vi "Export Strings.vi"(4 "error in":errorcluster, 5 "Log File":path, 6 "String File":path, 7 "Target":path) -> (0 "error out":errorcluster, 1 "Log File Out":path, 2 "String File Out":path)   [LabVIEW 2025]
doc: "This VI exports all strings of a single VI or of all elements in a LabVIEW Project to a file using the <b>VIs Strings.Export</b> invoke method. Additionally, the histories of all VIs and the descriptions of the project and of any libraries (classes) are added to the exported file.\n\nThe provided target <b>must</b> have the extension <i>.lvproj</i> or <i>.vi</i>.\n\nThe path input <b>Log File</b> is passed only to the <b>VIs Strings.Export</b> invoke method and has no further usage.\n\nThe <b>String File</b> and <b>Log File</b> inputs are optional. If they are not provided the files will be saved to a temporary location. The used paths are represented by the correspondent outputs."
uses:
  Type Definitions/Export Strings States--enum.ctl
  Type Definitions/Export Strings Data--enum.ctl
  Type Definitions/Extensions--enum.ctl
  Type Definitions/Project References--cluster.ctl
  <vilib>/Utility/EditLVProj/Library And VI References.ctl
  <userlib>/_OpenG.lib/file/file.llb/Strip Path Extension - Path__ogtk.vi
  <userlib>/_OpenG.lib/file/file.llb/Strip Path - Traditional__ogtk.vi
  <userlib>/_OpenG.lib/file/file.llb/File Exists - Scalar__ogtk.vi
  <vilib>/Utility/EditLVProj/Edit LVProj.lvlib
  <userlib>/_OpenG.lib/file/file.llb/openg_file.lvlib
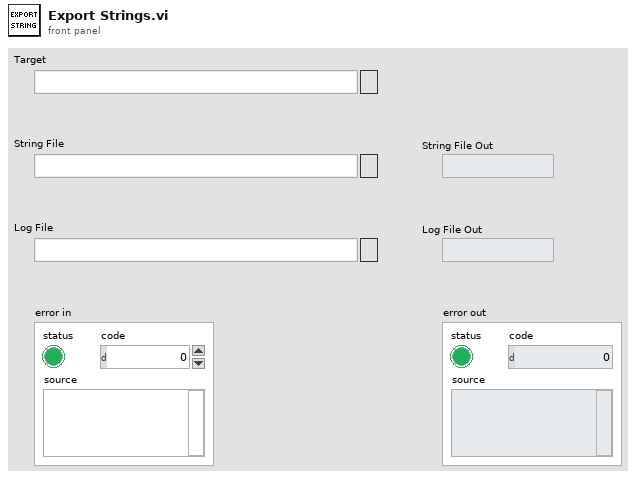
[diagram p1: front panel]
types:
  T1 = typedef "Export Strings Data--enum.ctl" = cluster{"Extension":T2, "String File":path, "Log File":path, "All VIs":refnum<vi>[], "All Libraries":refnum<vi>[], "Reference":variant}
  T2 = typedef "Extensions--enum.ctl" = enum16{"lvproj", "vi"}
  T3 = typedef "Export Strings States--enum.ctl" = enum16{"Initialize", "Exit", "Export Strings", "Export Project Desc.", "Remove Files", "Export VI Histories", "Export Libraries Desc.", "Prepare VI", "Prepare Project", "Create Folders"}
  T4 = typedef "Project References--cluster.ctl" = cluster{"Project Ref":refnum<vi>, "VI-Lib Ref":T5[]}
  T5 = typedef "Edit LVProj.lvlib/Library And VI References.ctl" = cluster{"Target Reference":refnum<vi>, "VI References":refnum<vi>[], "Library References":refnum<vi>[]}
  T6 = enum16{"open", "replace", "create", "open or create", "replace or create", "replace or create with confirmation"}
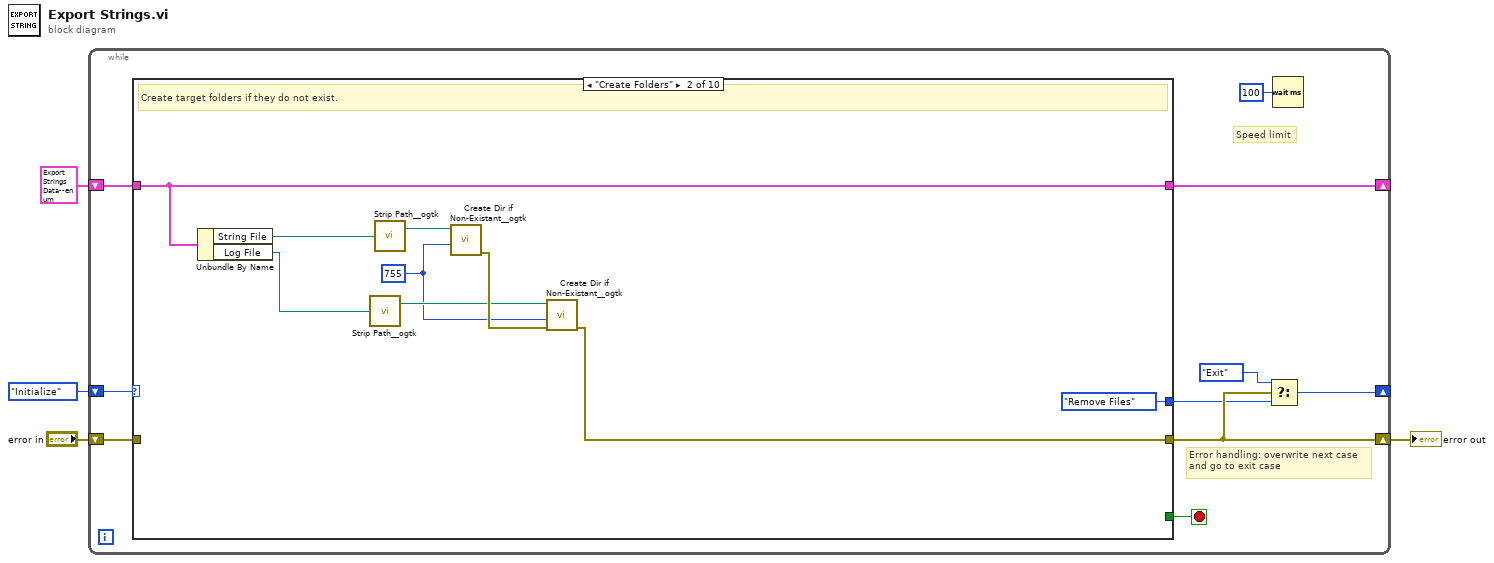
[diagram p0: block diagram]
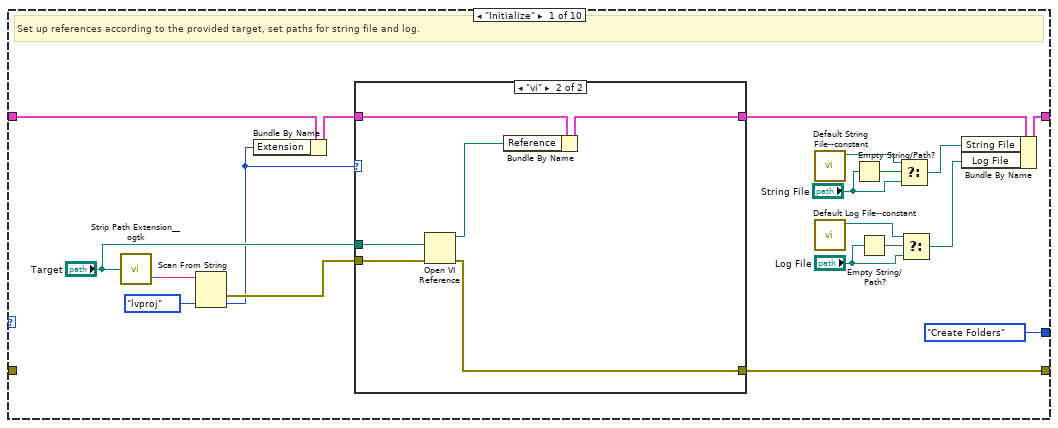
[diagram p2: hidden frame]
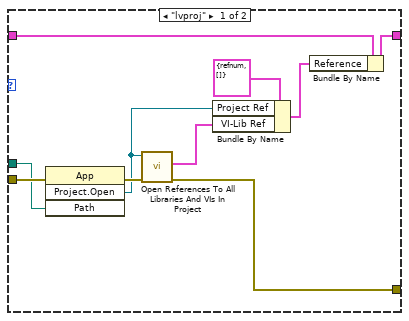
[diagram p3: hidden frame]
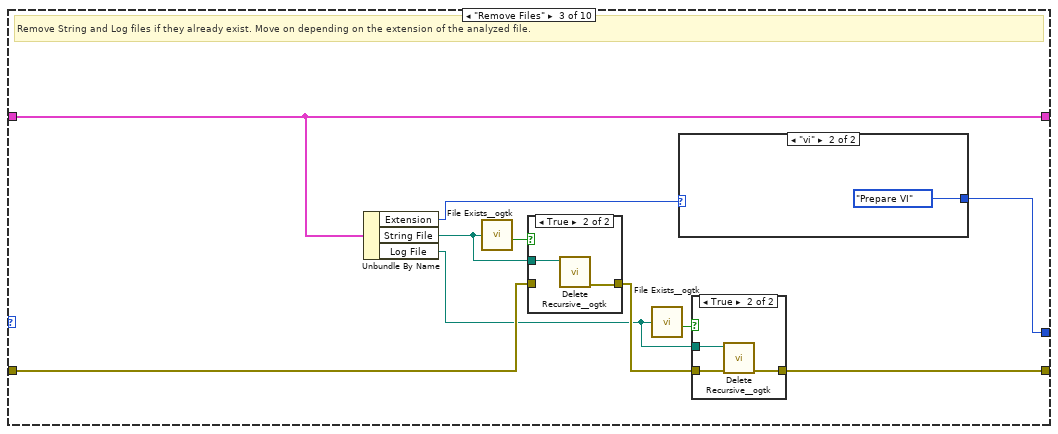
[diagram p4: hidden frame]
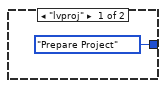
[diagram p5: hidden frame]
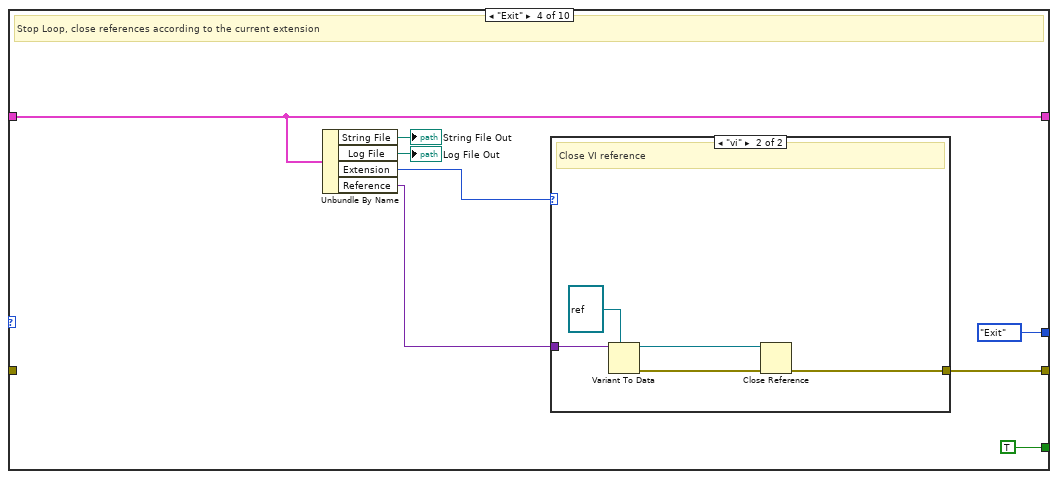
[diagram p8: hidden frame]
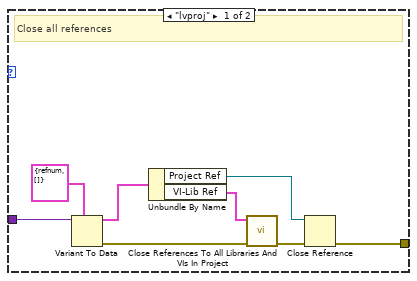
[diagram p9: hidden frame]
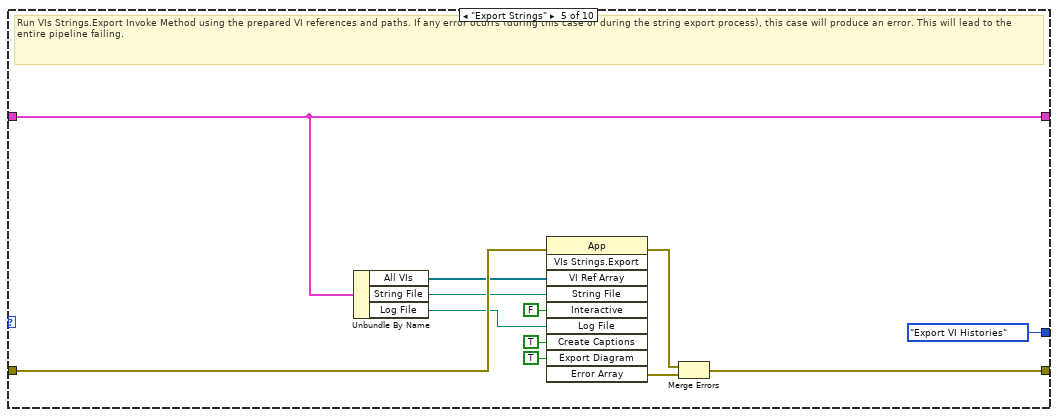
[diagram p10: hidden frame]
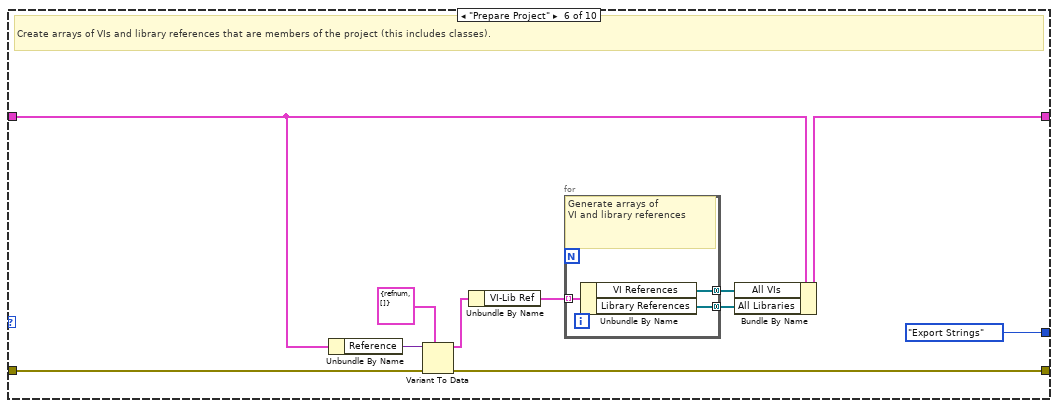
[diagram p11: hidden frame]
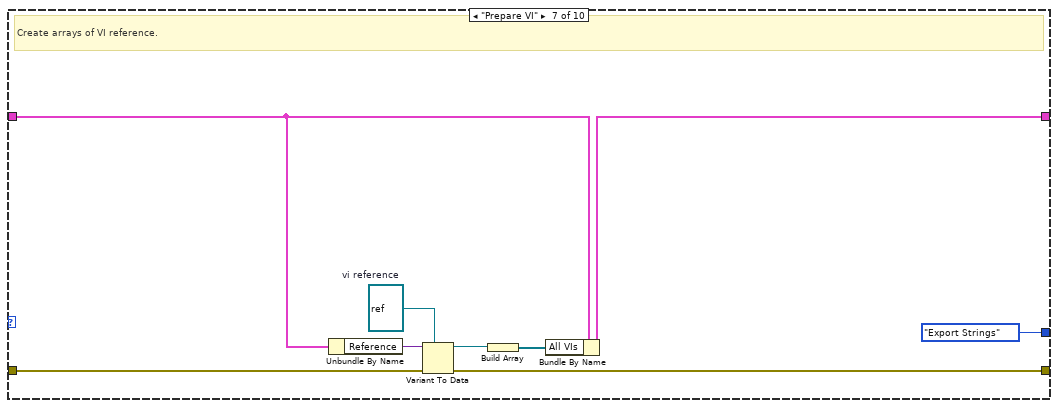
[diagram p12: hidden frame]
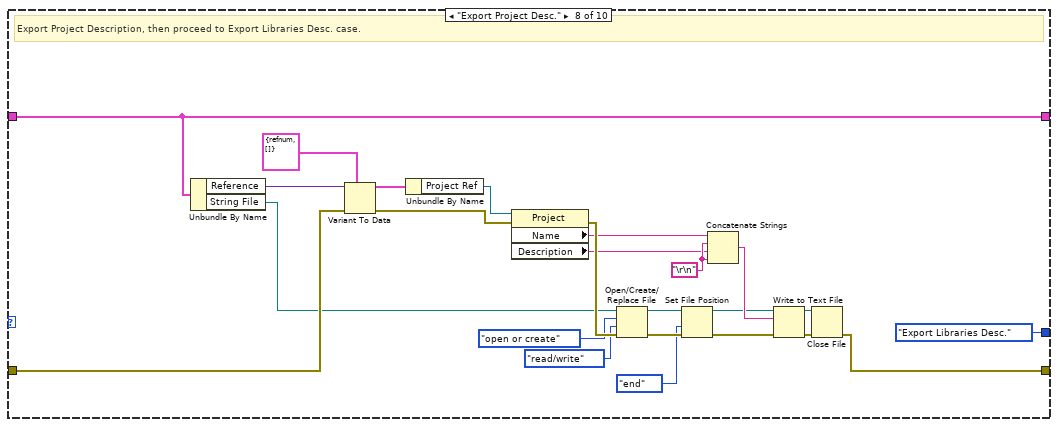
[diagram p13: hidden frame]
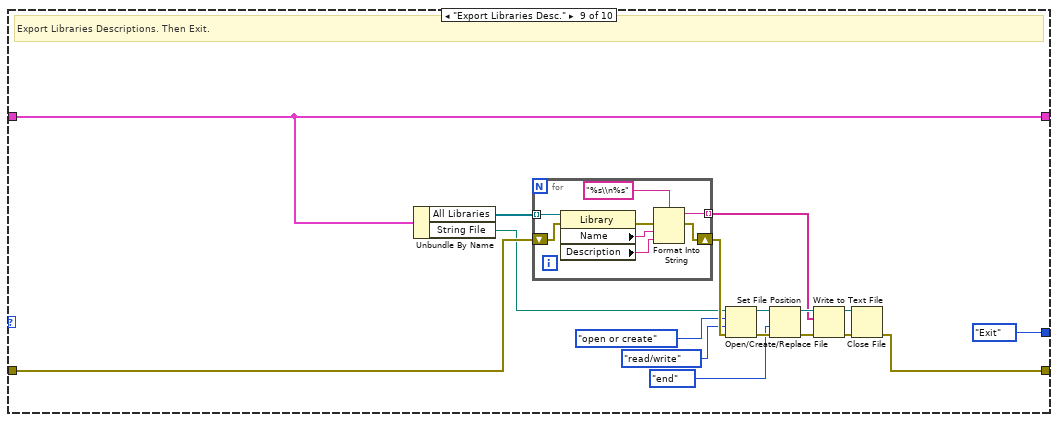
[diagram p14: hidden frame]
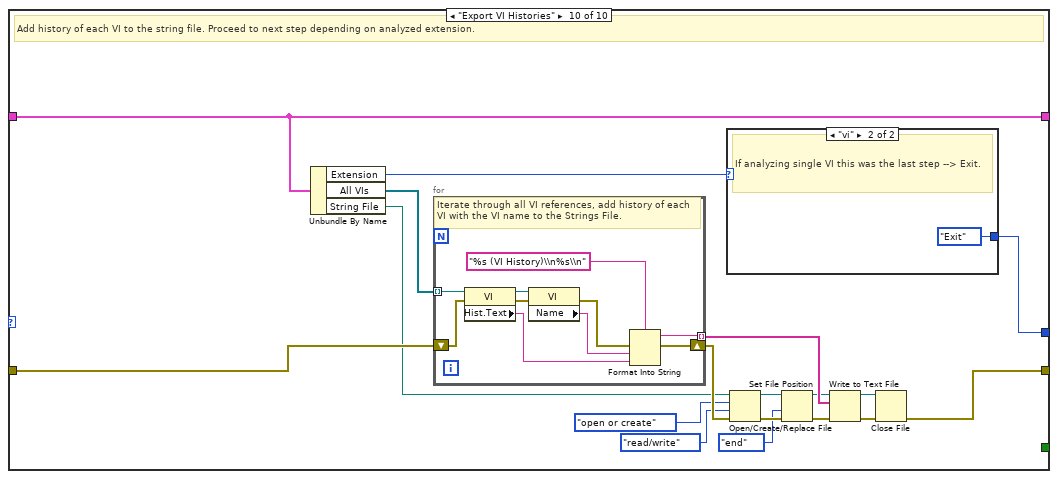
[diagram p15: hidden frame]
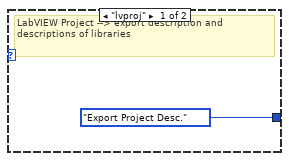
[diagram p16: hidden frame]
diagram:
  n1 = while {
    shift-right: [w8] -> _
    shift-left: Export_Strings_States--enum."Initialize" -> [w12]
    shift-right: [w14] -> w3
    shift-left: "error in" -> [w13]
    shift-right: [w6] -> _
    shift-left: T1 {"Extension"=enum."lvproj", "String File"=path "", "Log File"=path "", "All VIs"=[], "All Libraries"=[], "Reference"=variant} ("Export Strings Data") -> [w7]
    stop <- w11 stop-if-true
    # "Speed limit"
    # "Error handling: overwrite next case\nand go to exit case"
    n2 = case shown="\"Create Folders\"" w12 {
      tunnel: [_ _ _ TRUE _ _ _ _ _ _] -> w11
      tunnel: [w32 w57 w67 w85 w109 w120 w132 w157 w174 w200] -> w14
      tunnel: [Export_Strings_States--enum."Create Folders" Export_Strings_States--enum."Remove Files" w59 Export_Strings_States--enum."Exit" Export_Strings_States--enum."Export VI Histories" Export_Strings_States--enum."Export Strings" Export_Strings_States--enum."Export Strings" Export_Strings_States--enum."Export Libraries Desc." Export_Strings_States--enum."Exit" w183] -> w10
      tunnel: w13 -> [_ _ w66 _ w108 w121 w133 w151 w173 w196]
      tunnel: w7 -> [w16 w55 w65 w79 w99 w118 w130 w149 w167 w194]
      tunnel: [w22 w55 w65 w79 w99 w119 w131 w149 w167 w194] -> w6
      frame "Initialize" {
        # "Set up references according to the provided target, set paths for string file and log."
        n3 = call-poly <userlib>:"Strip Path Extension__ogtk.vi"("path"="Target") -> ("extension"=w30:string)  [unwired: 1 out]
        n4 = Scan From String(input string=w30, default 1=Extensions--enum."lvproj" ("Extensions")) -> (error out=w33:errorcluster, output 1=w15:T2)  [unwired: 3 in, 2 out]
        n5 = Bundle By Name(cluster=w16, "Extension"=w15) -> (w17:T1)
        n6 = case shown="\"vi\"" w15 {
          tunnel: w17 -> [w39 w44]
          tunnel: "Target" -> [w40 w47]
          tunnel: [w38 w45] -> w23
          tunnel: w33 -> [w42 w49]
          tunnel: [w41 w48] -> w32
          frame "lvproj" {
            n7 = invoke class="App" method="Project.Open"(error in=w42, "Path"=w40) -> (error out=w43:errorcluster, "Project:Open"=w36:refnum<vi>)  [unwired: 2 in, 2 out]
            n8 = call <vilib>:"Open References To All Libraries And VIs In Project.vi"("error in (no error)"=w43, "Project in"=w36) -> ("error out"=w41:errorcluster, "VI and Library References"=w35:T5[])  [unwired: 7 in, 1 out]
            n9 = Bundle By Name(cluster=T4 {"Project Ref"=refnum, "VI-Lib Ref"=[]} ("Project References"), "Project Ref"=w36, "VI-Lib Ref"=w35) -> (w34:T4)
            n10 = Bundle By Name(cluster=w39, "Reference"=w34) -> (w38:T1)
          }
          frame "vi" {
            n11 = Open VI Reference(vi path=w47, error in (no error)=w49) -> (vi reference=w46:refnum<vi>, error out=w48:errorcluster)  [unwired: 4 in]
            n12 = Bundle By Name(cluster=w44, "Reference"=w46) -> (w45:T1)
          }
        }
        n13 = call "Default String File--constant.vi"() -> ("Default String File"=w21:path)  [unwired: 7 in]
        n14 = call "Default Log File--constant.vi"() -> ("Default Log File"=w28:path)  [unwired: 7 in]
        n15 = Empty String/Path?(string/path="String File") -> (empty?=w26:bool)
        n16 = Empty String/Path?(string/path="Log File") -> (empty?=w27:bool)
        n17 = Select(t=w21, s=w26, f="String File") -> (s? t:f=w20:path)
        n18 = Select(t=w28, s=w27, f="Log File") -> (s? t:f=w19:path)
        n19 = Bundle By Name(cluster=w23, "String File"=w20, "Log File"=w19) -> (w22:T1)
      }
      frame "Create Folders" {
        w50 = i16 755 ("permissions (0755)")
        # "Create target folders if they do not exist."
        n20 = Unbundle By Name(w55) -> ("String File"=w54:path, "Log File"=w53:path)
        n21 = call-poly <userlib>:"Strip Path__ogtk.vi"("path"=w53) -> ("stripped path"=w51:path)  [unwired: 1 out]
        n22 = call-poly <userlib>:"Strip Path__ogtk.vi"("path"=w54) -> ("stripped path"=w52:path)  [unwired: 1 out]
        n23 = call <userlib>:"Create Dir if Non-Existant__ogtk.vi"("permissions (0755)"=w50, "Directory Path"=w52) -> ("error out"=w58:errorcluster)  [unwired: 7 in, 2 out]
        n24 = call <userlib>:"Create Dir if Non-Existant__ogtk.vi"("error in (no error)"=w58, "permissions (0755)"=w50, "Directory Path"=w51) -> ("error out"=w57:errorcluster)  [unwired: 6 in, 2 out]
      }
      frame "Remove Files" {
        # "Remove String and Log files if they already exist. Move on depending on the extension of the analyzed file."
        n25 = Unbundle By Name(w65) -> ("Extension"=w60:T2, "String File"=w63:path, "Log File"=w62:path)
        n26 = call-poly <userlib>:"File Exists__ogtk.vi"("file path"=w63) -> ("exists"=w64:bool)  [unwired: 6 in, 1 out]
        n27 = case shown="True" w64 {
          tunnel: w63 -> [_ w76]
          tunnel: [w75 w77] -> w68
          tunnel: w66 -> [w75 _]
          frame False {
          }
          frame True {
            n28 = call <userlib>:"Delete Recursive__ogtk.vi"("Path"=w76) -> ("error out"=w77:errorcluster)  [unwired: 9 in, 1 out]
          }
        }
        n29 = call-poly <userlib>:"File Exists__ogtk.vi"("file path"=w62) -> ("exists"=w61:bool)  [unwired: 6 in, 1 out]
        n30 = case shown="\"vi\"" w60 {
          tunnel: [Export_Strings_States--enum."Prepare Project" Export_Strings_States--enum."Prepare VI"] -> w59
          frame "lvproj" {
          }
          frame "vi" {
          }
        }
        n31 = case shown="True" w61 {
          tunnel: w62 -> [_ w72]
          tunnel: w68 -> [w71 w74]
          tunnel: [w71 w73] -> w67
          frame False {
          }
          frame True {
            n32 = call <userlib>:"Delete Recursive__ogtk.vi"("error in (no error)"=w74, "Path"=w72) -> ("error out"=w73:errorcluster)  [unwired: 8 in, 1 out]
          }
        }
      }
      frame "Exit" {
        # "Stop Loop, close references according to the current extension"
        n33 = Unbundle By Name(w79) -> ("String File"=→"String File Out":path, "Log File"=→"Log File Out":path, "Extension"=w80:T2, "Reference"=w78:variant)
        n34 = case shown="\"vi\"" w80 {
          tunnel: w78 -> [w90 w96]
          tunnel: [w92 w98] -> w85
          frame "lvproj" {
            # "Close all references"
            n35 = Variant To Data(type=T4 {"Project Ref"=refnum, "VI-Lib Ref"=[]} ("Project References"), Variant=w90) -> (data=w88:T4, error out=w91:errorcluster)  [unwired: 1 in]
            n36 = Unbundle By Name(w88) -> ("Project Ref"=w87:refnum<vi>, "VI-Lib Ref"=w86:T5[])
            n37 = call <vilib>:"Close References To All Libraries And VIs In Project.vi"("error in (no error)"=w91, "VI and Library References"=w86) -> ("error out"=w93:errorcluster)  [unwired: 9 in]
            n38 = Close Reference(reference=w87, error in (no error)=w93) -> (error out=w92:errorcluster)
          }
          frame "vi" {
            # "Close VI reference"
            n39 = Variant To Data(type=refnum<vi> refnum ("vi reference"), Variant=w96) -> (data=w94:refnum<vi>, error out=w97:errorcluster)  [unwired: 1 in]
            n40 = Close Reference(reference=w94, error in (no error)=w97) -> (error out=w98:errorcluster)
          }
        }
      }
      frame "Export Strings" {
        # "Run VIs Strings.Export Invoke Method using the prepared VI references and paths. If any error ocurrs (during this case or during the string export process), this case will produce an error. This will lead to the entire pipeline failing."
        n41 = Unbundle By Name(w99) -> ("All VIs"=w102:refnum<vi>[], "String File"=w101:path, "Log File"=w100:path)
        n42 = invoke class="App" method="VIs Strings.Export"(error in=w108, "VI Ref Array"=w102, "String File"=w101, "Interactive"=FALSE, "Log File"=w100, "Create Captions"=TRUE, "Export Diagram"=TRUE) -> (error out=w110:errorcluster, "Error Array"=w107:errorcluster[])  [unwired: 3 in, 8 out]
        n43 = Merge Errors(w110, w107) -> (w109:errorcluster)
      }
      frame "Prepare Project" {
        # "Create arrays of VIs and library references that are members of the project (this includes classes)."
        n44 = Unbundle By Name(w118) -> ("Reference"=w115:variant)
        n45 = Variant To Data(error in=w121, type=T4 {"Project Ref"=refnum, "VI-Lib Ref"=[]} ("Project References"), Variant=w115) -> (data=w112:T4, error out=w120:errorcluster)
        n46 = Unbundle By Name(w112) -> ("VI-Lib Ref"=w111:T5[])
        n47 = for {
          tunnel: w111 -> [w124] mode=indexing
          tunnel: [w123] -> w117 mode=concatenating
          tunnel: [w122] -> w116 mode=concatenating
          # "Generate arrays of\nVI and library references"
          n48 = Unbundle By Name(w124) -> ("VI References"=w123:refnum<vi>[], "Library References"=w122:refnum<vi>[])
        }
        n49 = Bundle By Name(cluster=w118, "All VIs"=w117, "All Libraries"=w116) -> (w119:T1)
      }
      frame "Prepare VI" {
        w127 = refnum<vi> refnum  # vi reference
        # "Create arrays of VI reference."
        n50 = Unbundle By Name(w130) -> ("Reference"=w129:variant)
        n51 = Variant To Data(error in=w133, type=w127, Variant=w129) -> (data=w126:refnum<vi>, error out=w132:errorcluster)
        n52 = Build Array(w126) -> (w125:refnum<vi>[])
        n53 = Bundle By Name(cluster=w130, "All VIs"=w125) -> (w131:T1)
      }
      frame "Export Project Desc." {
        w143 = "\r\n"
        # "Export Project Description, then proceed to Export Libraries Desc. case."
        n54 = Unbundle By Name(w149) -> ("Reference"=w136:variant, "String File"=w148:path)
        n55 = Variant To Data(error in=w151, type=T4 {"Project Ref"=refnum, "VI-Lib Ref"=[]} ("Project References"), Variant=w136) -> (data=w135:T4, error out=w152:errorcluster)
        n56 = Unbundle By Name(w135) -> ("Project Ref"=w134:refnum<vi>)
        n57 = property class="Project"(reference=w134, error in=w152) -> (error out=w156:errorcluster, "Name"=w142:string, "Description"=w141:string)  [unwired: 1 out]
        n58 = Open/Create/Replace File(file path (use dialog)=w148, error in=w156, operation (0:open)=T6."open or create", access (0:read/write)=enum16{"read/write", "read-only", "write-only"}."read/write") -> (refnum out=w140:refnum<file>, error out=w154:errorcluster)  [unwired: 2 in, 1 out]
        n59 = Set File Position(refnum=w140, from (0:start)=enum16{"start", "end", "current"}."end", error in=w154) -> (refnum out=w139:refnum<file>, error out=w153:errorcluster)  [unwired: 1 in]
        n60 = Concatenate Strings(w142, w143, w141, w143) -> (w145:string)
        n61 = Write to Text File(file (use dialog)=w139, text=w145, error in=w153) -> (refnum out=w144:refnum<file>, error out=w155:errorcluster)  [unwired: 1 in, 1 out]
        n62 = Close File(refnum=w144, error in=w155) -> (error out=w157:errorcluster)  [unwired: 1 out]
      }
      frame "Export Libraries Desc." {
        # "Export Libraries Descriptions. Then Exit."
        n63 = Unbundle By Name(w167) -> ("All Libraries"=w159:refnum<vi>[], "String File"=w166:path)
        n64 = for {
          tunnel: w159 -> [w179] mode=indexing
          tunnel: [w175] -> w158 mode=indexing
          shift-right: [w180] -> w169
          shift-left: w173 -> [w181]
          n65 = property class="Library"(reference=w179, error in=w181) -> (error out=w182:errorcluster, "Name"=w177:string, "Description"=w176:string)  [unwired: 1 out]
          n66 = Format Into String(format string="%s\\n%s", error in=w182, w177, w176) -> (resulting string=w175:string, error out=w180:errorcluster)  [unwired: 1 in]
        }
        n67 = Open/Create/Replace File(file path (use dialog)=w166, error in=w169, operation (0:open)=T6."open or create", access (0:read/write)=enum16{"read/write", "read-only", "write-only"}."read/write") -> (refnum out=w162:refnum<file>, error out=w171:errorcluster)  [unwired: 2 in, 1 out]
        n68 = Set File Position(refnum=w162, from (0:start)=enum16{"start", "end", "current"}."end", error in=w171) -> (refnum out=w161:refnum<file>, error out=w170:errorcluster)  [unwired: 1 in]
        n69 = Write to Text File(file (use dialog)=w161, text=w158, error in=w170) -> (refnum out=w163:refnum<file>, error out=w172:errorcluster)  [unwired: 1 in, 1 out]
        n70 = Close File(refnum=w163, error in=w172) -> (error out=w174:errorcluster)  [unwired: 1 out]
      }
      frame "Export VI Histories" {
        # "Add history of each VI to the string file. Proceed to next step depending on analyzed extension."
        n71 = Unbundle By Name(w194) -> ("Extension"=w184:T2, "All VIs"=w189:refnum<vi>[], "String File"=w193:path)
        n72 = for {
          tunnel: w189 -> [w208] mode=indexing
          tunnel: [w203] -> w188 mode=indexing
          shift-right: [w209] -> w195
          shift-left: w196 -> [w210]
          # "Iterate through all VI references, add history of each VI with the VI name to the Strings File."
          n73 = property class="VI"(reference=w208, error in=w210) -> (reference out=w207:refnum<vi>, error out=w212:errorcluster, "Hist.Text"=w204:string)
          n74 = property class="VI"(reference=w207, error in=w212) -> (error out=w211:errorcluster, "Name"=w205:string)  [unwired: 1 out]
          n75 = Format Into String(format string="%s (VI History)\\n%s\\n", error in=w211, w205, w204) -> (resulting string=w203:string, error out=w209:errorcluster)  [unwired: 1 in]
        }
        n76 = case shown="\"vi\"" w184 {
          tunnel: [Export_Strings_States--enum."Export Project Desc." Export_Strings_States--enum."Exit"] -> w183
          frame "lvproj" {
            # "LabVIEW Project --> export description and\ndescriptions of libraries"
          }
          frame "vi" {
            # "If analyzing single VI this was the last step --> Exit."
          }
        }
        n77 = Open/Create/Replace File(file path (use dialog)=w193, error in=w195, operation (0:open)=T6."open or create", access (0:read/write)=enum16{"read/write", "read-only", "write-only"}."read/write") -> (refnum out=w187:refnum<file>, error out=w198:errorcluster)  [unwired: 2 in, 1 out]
        n78 = Set File Position(refnum=w187, from (0:start)=enum16{"start", "end", "current"}."end", error in=w198) -> (refnum out=w185:refnum<file>, error out=w197:errorcluster)  [unwired: 1 in]
        n79 = Write to Text File(file (use dialog)=w185, text=w188, error in=w197) -> (refnum out=w190:refnum<file>, error out=w199:errorcluster)  [unwired: 1 in, 1 out]
        n80 = Close File(refnum=w190, error in=w199) -> (error out=w200:errorcluster)  [unwired: 1 out]
      }
    }
    n81 = Select(t=Export_Strings_States--enum."Exit", s=w14, f=w10) -> (s? t:f=w8:T3)
    n82 = Wait (ms)(milliseconds to wait=u32 100) -> ()  [unwired: 1 out]
  }
  "error out" <- w3
